vi "write to fifo.vi"(0 "pulse_gen_and_detect_p2p in":refnum<class "pulse_gen_and_detect_p2p.lvclass">, 11 "error in (no error)":errorcluster) -> (4 "pulse_gen_and_detect_p2p out":refnum<class "pulse_gen_and_detect_p2p.lvclass">, 6 "done write file":bool=TRUE, 8 "num of pulses sent to the FPGA":u32, 10 "room on fifo":bool=TRUE, 15 "error out":errorcluster)   [LabVIEW 2021, in "pulse_gen_and_detect_p2p.lvclass"]
uses:
  pulse_gen_and_detect_p2p.lvclass
  pulse_gen_and_detect_p2p.lvclass/pulse_gen_and_detect_p2p.ctl
  <vilib>/rvi/interface/nirviMethod/nirviMethod.xnode
  <vilib>/FPGAPlugInAG/Dynamic/niLvFpga_WriteFifo_Dynamic.vi
  <vilib>/rvi/errors/niLvFpgaMergeErrorWithErrorCode.vi
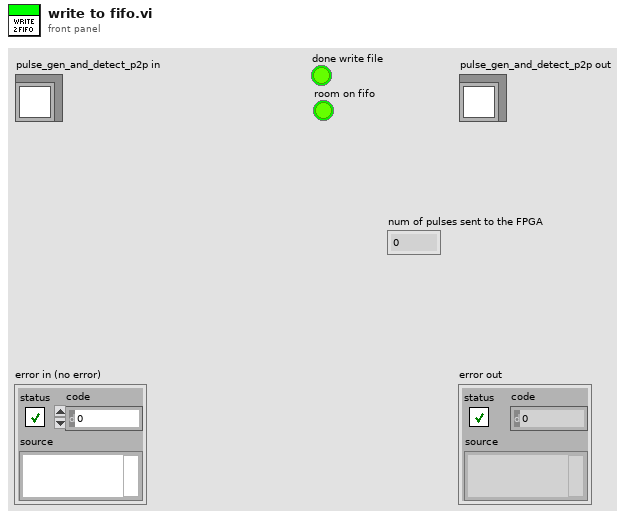
[diagram p1: front panel]
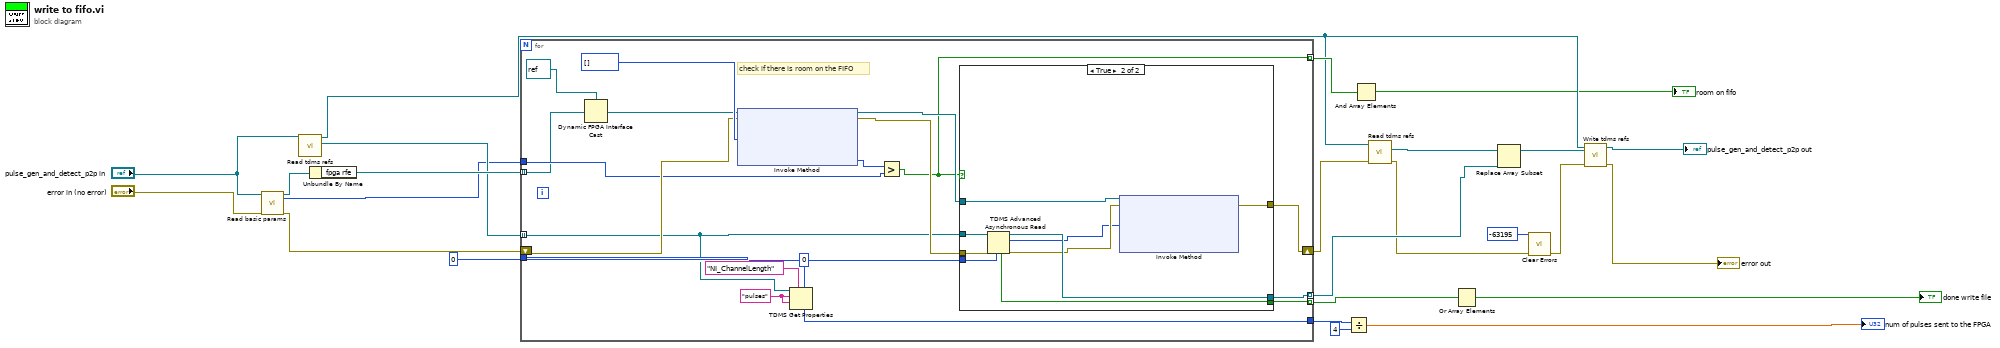
[diagram p0: block diagram]
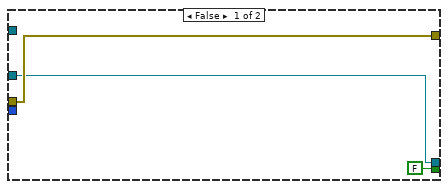
[diagram p2: hidden frame]
diagram:
  n1 = call-dynamic "Read basic params.vi"("device_type in"="pulse_gen_and_detect_p2p in", "error in (no error)"="error in (no error)") -> ("device_type out"=w15:refnum<class "pulse_gen_and_detect_p2p.lvclass">, "buffer size"=w16:u32, "error out"=w14:errorcluster)  [unwired: 12 in, 3 out]
  n2 = call-dynamic "Read tdms refs.vi"("device_type in"="pulse_gen_and_detect_p2p in") -> ("tdms refs"=w17:refnum<k34>[], "device_type out"=w12:refnum<class "pulse_gen_and_detect_p2p.lvclass">)  [unwired: 8 in, 1 out]
  n3 = Unbundle By Name(w15) -> ("fpga rfe"=w21:refnum<k20>[])
  n4 = for {
    tunnel: w17 -> [w27] mode=indexing
    tunnel: w21 -> [w33] mode=indexing
    tunnel: u64 0 ("type") -> [w44]
    tunnel: [w43] -> w22 mode=indexing
    tunnel: [w42] -> w18 mode=indexing
    shift-right: [w41] -> w6
    shift-left: w14 -> [w39]
    tunnel: [w26] -> w24
    tunnel: w16 -> [w38]
    tunnel: [w35] -> w19 mode=indexing
    w28 = "pulses" ("channel name")
    # "check if there is room on the FIFO"
    n5 = Dynamic FPGA Interface Cast(Session In=refnum<k20> refnum ("FPGA VI Reference Out"), Type=w33) -> (Session Out=w32:refnum<k20>)
    n6 = xnode "Invoke Method"("FPGA VI Reference In"=w32, "error in"=w39, "Data"=u64[] []) -> ("FPGA VI Reference Out"=w36:refnum<k20>, "error out"=w37:errorcluster, "Empty Elements Remaining"=w34:u32)  [unwired: 1 in]
    n7 = TDMS Get Properties(5:u64 0, 7:"NI_ChannelLength" ("property name"), 9:w28, 10:w28, 11:w27) -> (4:w26:u64)  [unwired: 1 in, 5 out]
    n8 = Greater?(x=w34, y=w38) -> (0:w35:bool)
    n9 = case shown="True" w35 {
      tunnel: w27 -> [w46 w56]
      tunnel: w44 -> [_ w55]
      tunnel: [FALSE ("read process finished?") w54] -> w43
      tunnel: [w46 w53] -> w42
      tunnel: [w47 w51] -> w41
      tunnel: w37 -> [w47 w49]
      tunnel: w36 -> [_ w48]
      frame False {
      }
      frame True {
        n10 = TDMS Advanced Asynchronous Read(6:w55, 8:w49, 11:w56) -> (0:w52:errorcluster, 2:w50:u64[], 3:w53:refnum<k34>, 4:w54:bool)
        n11 = xnode "Invoke Method"("FPGA VI Reference In"=w48, "error in"=w52, "Data"=w50) -> ("error out"=w51:errorcluster)  [unwired: 1 in, 2 out]
      }
    }
  }
  n12 = Divide(x=w24, y=4) -> (x/y=→"num of pulses sent to the FPGA":dbl)
  n13 = And Array Elements(Boolean array=w19) -> (logical AND=→"room on fifo":bool)
  n14 = call-dynamic "Read tdms refs.vi"("error in (no error)"=w6, "device_type in"=w12) -> ("error out"=w5:errorcluster, "tdms refs"=w13:refnum<k34>[])  [unwired: 7 in, 1 out]
  n15 = Or Array Elements(Boolean array=w22) -> (logical OR=→"done write file":bool)
  n16 = Replace Array Subset(array=w13, new element=w18) -> (w11:refnum<k34>[])  [unwired: 1 in]
  n17 = call <vilib>:"Clear Errors.vi"("error in (no error)"=w5, "specific error code to clear (0: all)"=-63195) -> ("error out"=w4:errorcluster)  [unwired: 4 in, 1 out]
  n18 = call-dynamic "Write tdms refs.vi"("error in (no error)"=w4, "tdms refs"=w11, "device_type in"=w12) -> ("error out"=→"error out":errorcluster, "device_type out"=→"pulse_gen_and_detect_p2p out":refnum<class "pulse_gen_and_detect_p2p.lvclass">)  [unwired: 7 in]
